vi "Get Kasli Index.vi"(8 "error in (no error)":errorcluster, 9 "Parallel?":bool, 10 "Schedule Block":refnum<class "Schedule Block.lvclass">=refnum, 11 "Scheduler in":refnum<class "Scheduler.lvclass">=refnum) -> (0 "error out":errorcluster, 2 "Index":i32, 3 "Scheduler out":refnum<class "Scheduler.lvclass">)   [LabVIEW 2020, in "CIRCUS_uServices.lvlib" / "Scheduler.lvlib" / "Scheduler.lvclass"]
uses:
  Scheduler.lvclass
  Run Utilities/Schedule Block/Schedule Block.lvclass
  e725186a-174a-45a5-83e2-4895d97151a7.vi
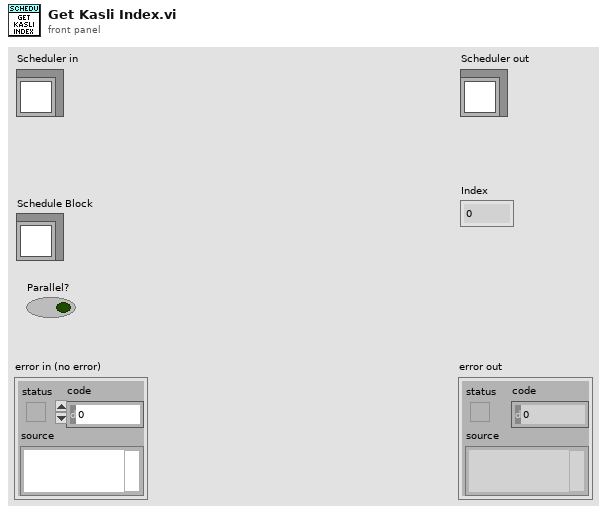
[diagram p1: front panel]
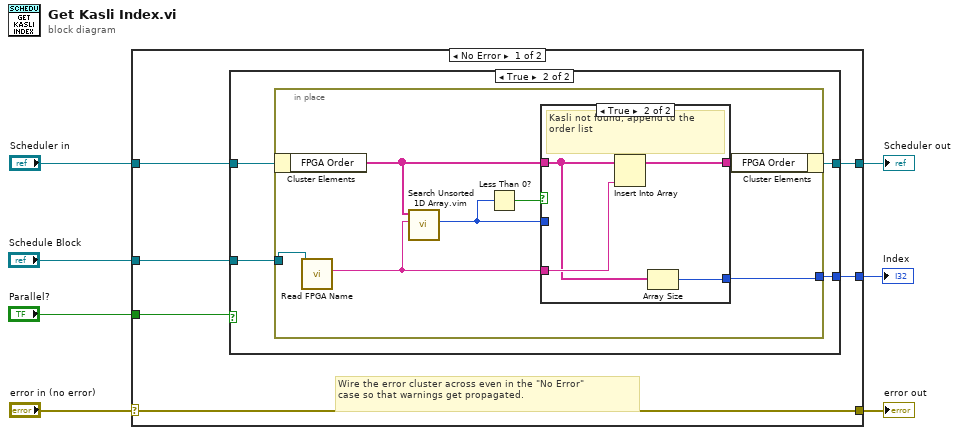
[diagram p0: block diagram]
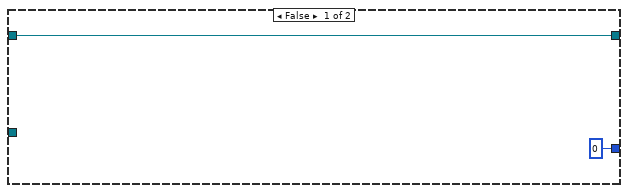
[diagram p2: hidden frame]
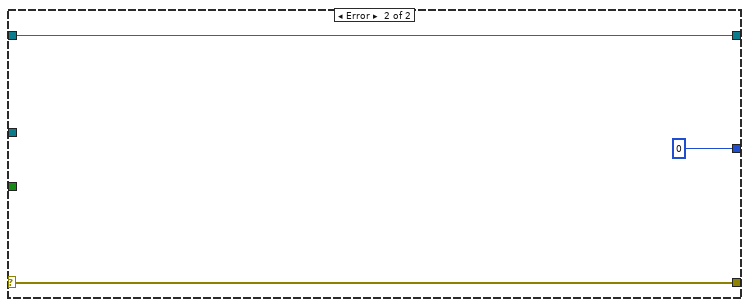
[diagram p4: hidden frame]
diagram:
  n1 = case shown="No Error" "error in (no error)" {
    selector: "error in (no error)" -> [w13 w35]
    tunnel: [w13 w35] -> w6
    tunnel: [w8 w34] -> w4
    tunnel: "Scheduler in" -> [w12 w34]
    tunnel: "Schedule Block" -> [w11 _]
    tunnel: [w10 0] -> w2
    tunnel: "Parallel?" -> [w9 _]
    frame No Error {
      # "Wire the error cluster across even in the \"No Error\"\ncase so that warnings get propagated."
      n2 = case shown="True" w9 {
        tunnel: w12 -> [w15 w17]
        tunnel: w11 -> [_ w19]
        tunnel: [0 w18] -> w10
        tunnel: [w15 w16] -> w8
        frame False {
        }
        frame True {
          n3 = in-place {
            in-place-border: w19 -> [w24]
            in-place-border: [w25] -> w18
            n4 = in-place-cluster #1(w17) -> ("FPGA Order"=w23:string[])
            n5 = call-dynamic "Read FPGA Name.vi"("Schedule Block in"=w24) -> ("FPGA Name"=w22:string)  [unwired: 8 in, 2 out]
            n6 = call "Search Unsorted 1D Array.vim"("element"=w22, "unsorted 1D array"=w23) -> ("index of element"=w20:i32)  [unwired: 9 in]
            n7 = Less Than 0?(x=w20) -> (x < 0?=w21:bool)
            n8 = case shown="True" w21 {
              tunnel: w23 -> [w28 w30]
              tunnel: [w28 w32] -> w26
              tunnel: w20 -> [w27 _]
              tunnel: [w27 w29] -> w25
              tunnel: w22 -> [_ w31]
              frame False {
                # "Found this Kasli, do nothing"
              }
              frame True {
                # "Kasli not found, append to the order list"
                n9 = Insert Into Array(array=w30, new element=w31) -> (w32:string[])  [unwired: 1 in]
                n10 = Array Size(array=w30) -> (size(s)=w29:i32)
              }
            }
            n11 = in-place-cluster #1("FPGA Order"=w26) -> (w16:refnum<class "Scheduler.lvclass">)
          }
        }
      }
    }
    frame Error {
    }
  }
  "error out" <- w6
  "Scheduler out" <- w4
  "Index" <- w2
